vi "_unittest Variant to String.vi"(8 "error in (no error)":errorcluster, 11 "Actual Value":variant) -> (0 "error out":errorcluster, 2 "Label":string, 3 "String":string)   [LabVIEW 2019, in "labview_json_tests.lvlib"]
uses:
  labview_json_tests.lvlib
  <vilib>/Utility/Data Type/NI_Data Type.lvlib
  lib/labview_json.lvlib
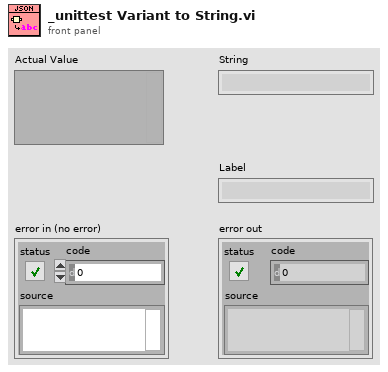
[diagram p1: front panel]
types:
  T1 = typedef "NI_Data Type.lvlib/Data Type.ctl" = enum8{"Invalid Type", "Void", "I8", "I16", "I32", "I64", "U8", "U16", "U32", "U64", "Single Float", "Double Float", "Extended Float", "Single Complex", "Double Complex", "Extended Complex", "Enum U8", "Enum U16", "Enum U32", "Enum U64", "Single Float With Unit", "Double Float With Unit", "Extended Float With Unit", "Single Complex with Unit", "Double Complex with Unit", "Extended Complex with Unit", "Boolean", "String", "Path", "Picture", "Tag", "Array", "Cluster", "Variant", "LV Variant", "Waveform", "Timestamp", "Digital Waveform", "Digital Data", "ExpressData", "Refnum", "External Data", "VI", "Poly VI", "LabVIEW Class Instance", "Fixed Point", "Set Collection", "Map Collection"}
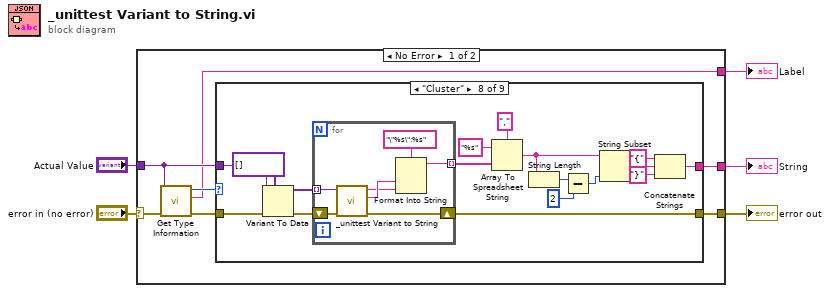
[diagram p0: block diagram]
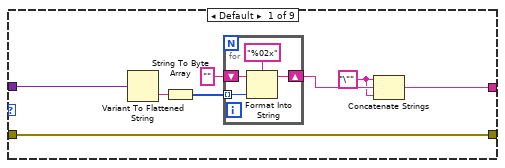
[diagram p2: hidden frame]
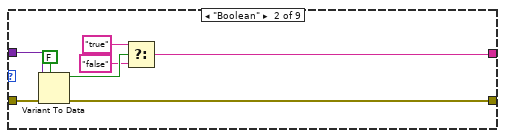
[diagram p3: hidden frame]
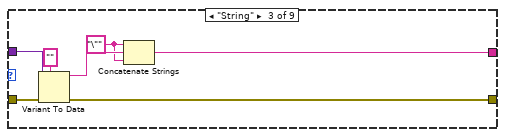
[diagram p4: hidden frame]
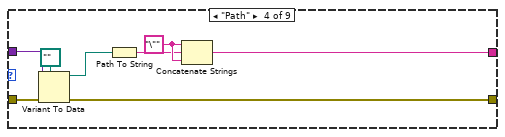
[diagram p5: hidden frame]
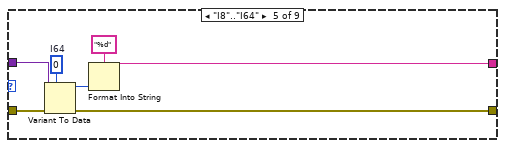
[diagram p6: hidden frame]
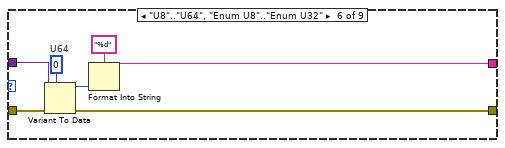
[diagram p7: hidden frame]
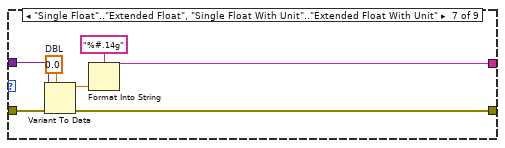
[diagram p8: hidden frame]
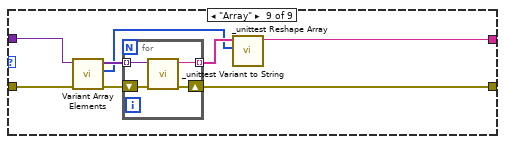
[diagram p9: hidden frame]
diagram:
  n1 = case shown="No Error" "error in (no error)" {
    selector: "error in (no error)" -> [w9 w105]
    tunnel: "Actual Value" -> [w10 _]
    tunnel: [w8 w105] -> w3
    tunnel: [w7 _] -> w2
    tunnel: [w6 _] -> w1
    frame No Error {
      n2 = call <vilib>:"Get Type Information.vi"("error in (no error)"=w9, "variant"=w10) -> ("error out"=w12:errorcluster, "name"=w7:string, "type"=w11:T1)  [unwired: 5 in, 2 out]
      n3 = case shown="\"Cluster\"" w11 {
        tunnel: w12 -> [w15 w32 w39 w47 w54 w61 w68 w85 w97]
        tunnel: w10 -> [w20 w30 w37 w45 w52 w59 w66 w84 w96]
        tunnel: [w15 w31 w38 w46 w53 w60 w67 w73 w100] -> w8
        tunnel: [w14 w26 w34 w42 w48 w55 w62 w71 w98] -> w6
        frame Default {
          w13 = "\"" ("string")
          n4 = Variant To Flattened String(Variant=w20) -> (data string=w17:string)  [unwired: 1 out]
          n5 = String To Byte Array(string=w17) -> (unsigned byte array=w19:u8[])
          n6 = for {
            tunnel: w19 -> [w24] mode=indexing
            shift-right: [w22] -> w16
            shift-left: "" -> [w21]
            n7 = Format Into String(format string="%02x", initial string=w21, w24) -> (resulting string=w22:string)  [unwired: 1 in, 1 out]
          }
          n8 = Concatenate Strings(w13, w16, w13) -> (w14:string)
        }
        frame "Boolean" {
          n9 = Variant To Data(error in=w32, type=FALSE, Variant=w30) -> (data=w28:bool, error out=w31:errorcluster)
          n10 = Select(t="true", s=w28, f="false") -> (s? t:f=w26:string)
        }
        frame "String" {
          w33 = "\"" ("string")
          n11 = Variant To Data(error in=w39, type="", Variant=w37) -> (data=w35:string, error out=w38:errorcluster)
          n12 = Concatenate Strings(w33, w35, w33) -> (w34:string)
        }
        frame "Path" {
          w41 = "\"" ("string")
          n13 = Variant To Data(error in=w47, type=path "", Variant=w45) -> (data=w43:path, error out=w46:errorcluster)
          n14 = Path To String(path=w43) -> (string=w40:string)
          n15 = Concatenate Strings(w41, w40, w41) -> (w42:string)
        }
        frame "I8".."I64" {
          w51 = i64 0  # I64
          n16 = Variant To Data(error in=w54, type=w51, Variant=w52) -> (data=w50:i64, error out=w53:errorcluster)
          n17 = Format Into String(format string="%d", w50) -> (resulting string=w48:string)  [unwired: 2 in, 1 out]
        }
        frame "U8".."U64", "Enum U8".."Enum U32" {
          w58 = u64 0  # U64
          n18 = Variant To Data(error in=w61, type=w58, Variant=w59) -> (data=w57:u64, error out=w60:errorcluster)
          n19 = Format Into String(format string="%d", w57) -> (resulting string=w55:string)  [unwired: 2 in, 1 out]
        }
        frame "Single Float".."Extended Float", "Single Float With Unit".."Extended Float With Unit" {
          w65 = 0.0  # DBL
          n20 = Variant To Data(error in=w68, type=w65, Variant=w66) -> (data=w64:dbl, error out=w67:errorcluster)
          n21 = Format Into String(format string="%#.14g", w64) -> (resulting string=w62:string)  [unwired: 2 in, 1 out]
        }
        frame "Cluster" {
          n22 = Variant To Data(error in=w85, type=variant[] [], Variant=w84) -> (data=w81:variant[], error out=w82:errorcluster)
          n23 = for {
            tunnel: w81 -> [w91] mode=indexing
            tunnel: [w87] -> w80 mode=indexing
            shift-right: [w86] -> w73
            shift-left: w82 -> [w92]
            n24 = call "_unittest Variant to String.vi"("error in (no error)"=w92, "Actual Value"=w91) -> ("error out"=w86:errorcluster, "Label"=w90:string, "String"=w89:string)  [unwired: 7 in]
            n25 = Format Into String(format string="\"%s\":%s", w90, w89) -> (resulting string=w87:string)  [unwired: 2 in, 1 out]
          }
          n26 = Array To Spreadsheet String(delimiter (Tab)=",", array=w80, 3:"%s" ("format string")) -> (spreadsheet string=w77:string)
          n27 = String Length(string=w77) -> (length=w76:i32)
          n28 = Subtract(x=w76, y=2) -> (x-y=w74:i32)
          n29 = String Subset(string=w77, length (rest)=w74) -> (substring=w72:string)  [unwired: 1 in]
          n30 = Concatenate Strings("{" ("string"), w72, "}" ("string")) -> (w71:string)
        }
        frame "Array" {
          n31 = call "Variant Array Elements.vi"("error in (no error)"=w97, "N Dim Array"=w96) -> ("error out"=w95:errorcluster, "Sizes"=w93:i32[], "Elements"=w94:variant[])  [unwired: 6 in, 1 out]
          n32 = for {
            tunnel: w94 -> [w102] mode=indexing
            tunnel: [w101] -> w99 mode=indexing
            shift-right: [w103] -> w100
            shift-left: w95 -> [w104]
            n33 = call "_unittest Variant to String.vi"("error in (no error)"=w104, "Actual Value"=w102) -> ("error out"=w103:errorcluster, "String"=w101:string)  [unwired: 7 in, 1 out]
          }
          n34 = call "_unittest Reshape Array.vi"("Sizes"=w93, "Array Elements"=w99) -> ("String"=w98:string)  [unwired: 9 in]
        }
      }
    }
    frame Error {
    }
  }
  "String" <- w1
  "Label" <- w2
  "error out" <- w3
